vi "send.vi"(0 "object in":refnum<class "tcp_work.lvclass">, 1 "写入缓冲区":string, 5 "error in (no error)":errorcluster) -> (14 "object out":refnum<class "tcp_work.lvclass">, 19 "error out":errorcluster)   [LabVIEW 2016, in "tcp_work.lvclass"]
uses:
  tcp_work.lvclass
  tcp_work.lvclass/tcp_work.ctl
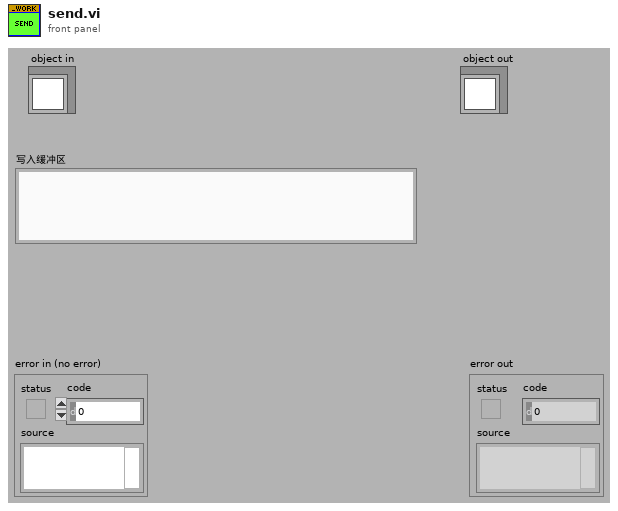
[diagram p1: front panel]
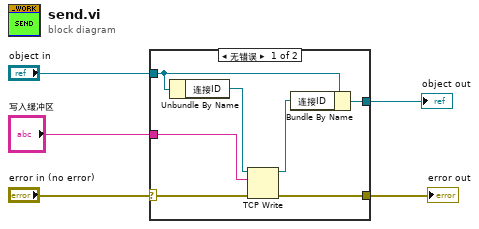
[diagram p0: block diagram]
diagram:
  n1 = case shown="无错误" "error in (no error)" {
    selector: "error in (no error)" -> [w7 w14]
    tunnel: [w6 w14] -> w4
    tunnel: [w11 w13] -> w2
    tunnel: "object in" -> [w12 w13]
    tunnel: "写入缓冲区" -> [w10 _]
    frame No Error {
      n2 = Unbundle By Name(w12) -> ("连接ID"=w9:refnum<k5>)
      n3 = TCP Write(connection ID=w9, data in=w10, error in (no error)=w7) -> (connection ID out=w8:refnum<k5>, error out=w6:errorcluster)  [unwired: 1 in, 1 out]
      n4 = Bundle By Name(cluster=w12, "连接ID"=w8) -> (w11:refnum<class "tcp_work.lvclass">)
    }
    frame Error {
    }
  }
  "error out" <- w4
  "object out" <- w2
